vi "getWaypoints.vi"(8 "Error In":errorcluster, 10 "NotifierReff 2":T1, 11 "RoundBouy in":refnum<class "RoundBouy.lvclass">) -> (0 "Error Out":errorcluster, 2 "Waypoint Array":refnum<class "Waypoint.lvclass">[](array[class]), 3 "RoundBouy out":refnum<class "RoundBouy.lvclass">)   [LabVIEW 2013, in "RoundBouy.lvclass"]
doc: "Generate and get the critical waypoints. In this case, at least two are generated, with a third dependent on where the next mission is. These also depend on which direction around the buoy the boat is going."
uses:
  RoundBouy.lvclass
  Waypoint/Waypoint.lvclass
  Data/TypeDefs/Notifiers.ctl
  Data/TypeDefs/UTM Location.ctl
  Data/TypeDefs/Sail Set Suggestions.ctl
  Data/TypeDefs/Rudder Set Suggestions.ctl
  Data/TypeDefs/OverrideInformation.ctl
  Data/TypeDefs/OverrideMode.ctl
  Data/TypeDefs/MotorSetup.ctl
  Data/TypeDefs/DynamixelSetupInfo.ctl
  Data/TypeDefs/AirmarStatus.ctl
  Data/TypeDefs/HardwareOnline.ctl
  Data/TypeDefs/DynamixelCycleTracker.ctl
  Data/TypeDefs/RC Input Values.ctl
  GenericMission/GenericMission.lvclass
  RoundBouy.lvclass/RoundBouy.ctl
  <vilib>/Analysis/coordinate.llb/2D Cartesian Coordinate Shift (Scalar).vi
  <vilib>/Analysis/coordinate.llb/2D Cartesian Coordinate Rotation (Scalar).vi
  <vilib>/Analysis/NI_AALPro.lvlib
panel:
  out "Mission X":dbl
  out "Mission Y":dbl
  out "wp1 Y":dbl
  out "wp1 X":dbl
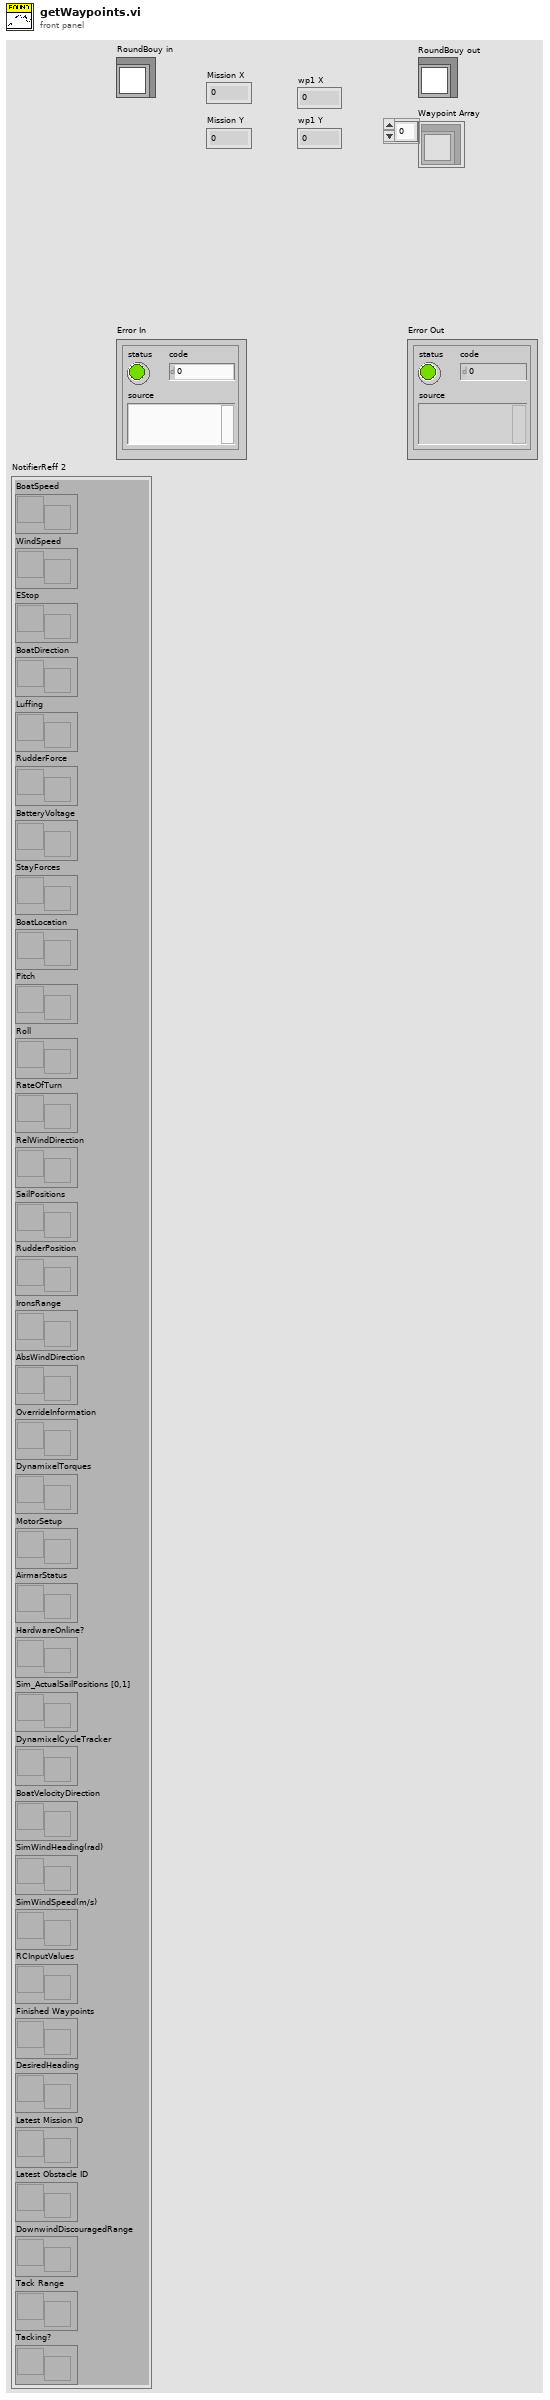
[diagram p1: front panel]
types:
  T1 = typedef "Notifiers.ctl" = cluster{"BoatSpeed":refnum<notifier>, "WindSpeed":refnum<notifier>, "EStop":refnum<notifier>, "BoatDirection":refnum<notifier>, "Luffing":refnum<notifier>, "RudderForce":refnum<notifier>, "BatteryVoltage":refnum<notifier>, "StayForces":refnum<notifier>, "BoatLocation":refnum<notifier>, "Pitch":refnum<notifier>, "Roll":refnum<notifier>, "RateOfTurn":refnum<notifier>, "RelWindDirection":refnum<notifier>, "SailPositions":refnum<notifier>, "RudderPosition":refnum<notifier>, "IronsRange":refnum<notifier>, "AbsWindDirection":refnum<notifier>, "OverrideInformation":refnum<notifier>, "DynamixelTorques":refnum<notifier>, "MotorSetup":refnum<notifier>, "AirmarStatus":refnum<notifier>, "HardwareOnline?":refnum<notifier>, "Sim_ActualSailPositions [0,1]":refnum<notifier>, "DynamixelCycleTracker":refnum<notifier>, "BoatVelocityDirection":refnum<notifier>, "SimWindHeading(rad)":refnum<notifier>, "SimWindSpeed(m/s)":refnum<notifier>, "RCInputValues":refnum<notifier>, "Finished Waypoints":refnum<notifier>, "DesiredHeading":refnum<notifier>, "Latest Mission ID":refnum<notifier>, "Latest Obstacle ID":refnum<notifier>, "DownwindDiscouragedRange":refnum<notifier>, "Tack Range":refnum<notifier>, "Tacking?":refnum<notifier>}
  T2 = typedef "UTM Location.ctl" = cluster{"UTM Zone":dbl, "Hemisphere":enum16{"North", "South"}, "East":dbl, "North":dbl}
  T3 = typedef "MissionTypeControl.ctl" = enum16{"Idle at Point", "Drive to Waypoint", "Round Buoy to Port", "Round Buoy to Starboard", "Pass Between Buoys", "Station Keeping"}
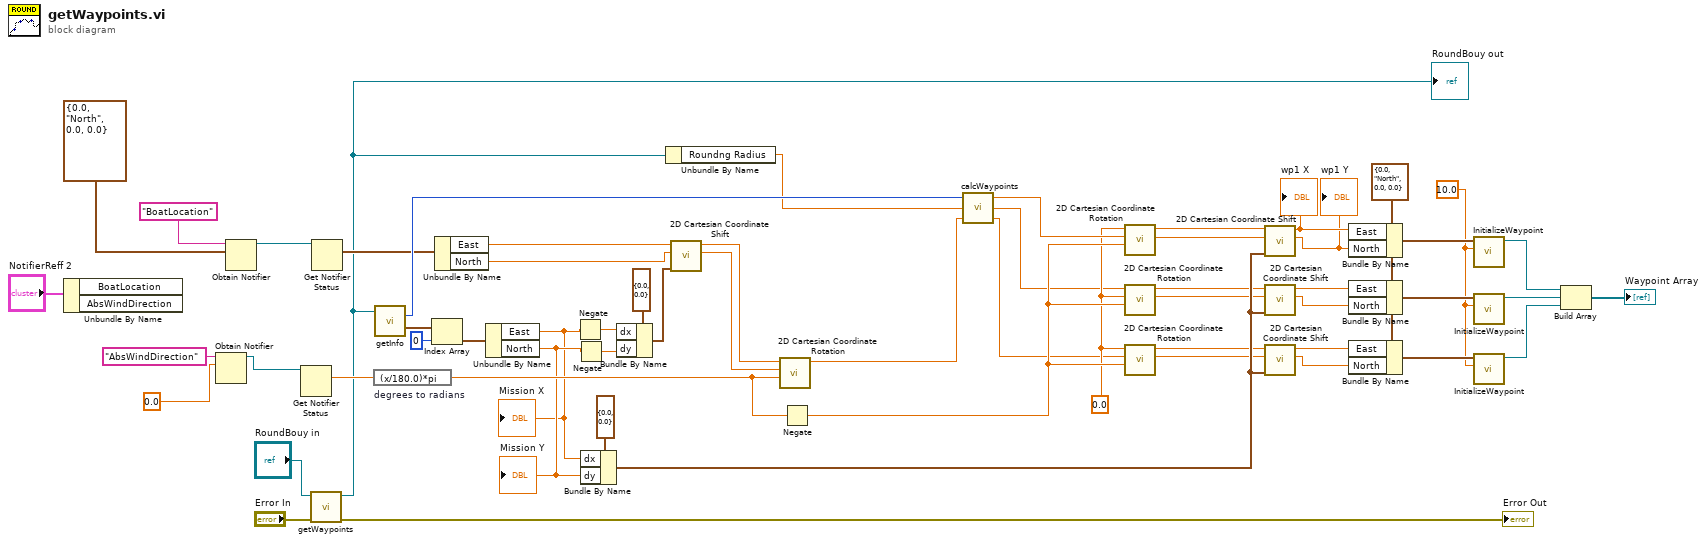
[diagram p0: block diagram]
diagram:
  w12 = 10.0
  w40 = 0.0 ("East")
  w44 = T2 {"UTM Zone"=0.0, "Hemisphere"=enum."North", "East"=0.0, "North"=0.0} ("Coords")
  n1 = Unbundle By Name("NotifierReff 2") -> ()  [unwired: 2 out]
  n2 = Obtain Notifier(name (unnamed)="AbsWindDirection", notification data type=0.0 ("latest notification")) -> (notifier out=w13:refnum<notifier>)  [unwired: 2 in, 2 out]
  n3 = Obtain Notifier(name (unnamed)="BoatLocation", notification data type=T2 {"UTM Zone"=0.0, "Hemisphere"=enum."North", "East"=0.0, "North"=0.0} ("latest notification")) -> (notifier out=w19:refnum<notifier>)  [unwired: 2 in, 2 out]
  n4 = Get Notifier Status(notifier=w13) -> (current notification=w11:dbl)  [unwired: 1 in, 4 out]
  n5 = call-parent "getWaypoints.vi"("Error In"="Error In", "GenericMission in"="RoundBouy in") -> ("Error Out"=→"Error Out":errorcluster, "GenericMission out"=w2:refnum<class "RoundBouy.lvclass">)  [unwired: 7 in, 1 out]
  "RoundBouy out" <- w2
  n6 = Get Notifier Status(notifier=w19) -> (current notification=w16:T2)  [unwired: 1 in, 4 out]
  n7 = expression code="(x/180.0)*pi" "degrees to radians"(w11) -> (w10:dbl)
  n8 = call-dynamic "getInfo.vi"("GenericMission in"=w2) -> ("Mission Type"=w43:T3, "Points of Interest"=w55:T2[])  [unwired: 6 in, 7 out]
  n9 = Index Array(array=w55, index=0) -> (element=w53:T2)
  n10 = Unbundle By Name(w16) -> ("East"=w8:dbl, "North"=w9:dbl)
  n11 = Unbundle By Name(w53) -> ("East"=w3:dbl, "North"=w4:dbl)
  "Mission Y" <- w4
  "Mission X" <- w3
  n12 = Negate(x=w3) -> (-x=w6:dbl)
  n13 = Negate(x=w4) -> (-x=w5:dbl)
  n14 = Bundle By Name(cluster=cluster{"dx":dbl, "dy":dbl} {"dx"=0.0, "dy"=0.0} ("shift"), "dx"=w3, "dy"=w4) -> (w36:cluster{"dx":dbl, "dy":dbl})
  n15 = Bundle By Name(cluster=cluster{"dx":dbl, "dy":dbl} {"dx"=0.0, "dy"=0.0} ("shift"), "dx"=w6, "dy"=w5) -> (w51:cluster{"dx":dbl, "dy":dbl})
  n16 = Unbundle By Name(w2) -> ("Roundng Radius"=w1:dbl)
  n17 = call-poly <vilib>:"2D Cartesian Coordinate Shift.vi"("shift"=w51, "y"=w9, "x"=w8) -> ("y out"=w50:dbl, "x out"=w49:dbl)  [unwired: 6 in, 1 out]
  n18 = call-poly <vilib>:"2D Cartesian Coordinate Rotation.vi"("theta"=w10, "y"=w50, "x"=w49) -> ("x out"=w7:dbl)  [unwired: 6 in, 2 out]
  n19 = Negate(x=w10) -> (-x=w41:dbl)
  n20 = call "calcWaypoints.vi"("boat x"=w7, "Clearance"=w1, "Mission Type"=w43) -> ("y 3"=w38:dbl, "x 2"=w39:dbl, "y 1"=w42:dbl)
  n21 = call-poly <vilib>:"2D Cartesian Coordinate Rotation.vi"("theta"=w41, "y"=w42, "x"=w40) -> ("y out"=w34:dbl, "x out"=w35:dbl)  [unwired: 6 in, 1 out]
  n22 = call-poly <vilib>:"2D Cartesian Coordinate Rotation.vi"("theta"=w41, "y"=w40, "x"=w39) -> ("y out"=w32:dbl, "x out"=w33:dbl)  [unwired: 6 in, 1 out]
  n23 = call-poly <vilib>:"2D Cartesian Coordinate Rotation.vi"("theta"=w41, "y"=w38, "x"=w40) -> ("y out"=w30:dbl, "x out"=w31:dbl)  [unwired: 6 in, 1 out]
  n24 = call-poly <vilib>:"2D Cartesian Coordinate Shift.vi"("shift"=w36, "y"=w34, "x"=w35) -> ("y out"=w28:dbl, "x out"=w29:dbl)  [unwired: 6 in, 1 out]
  "wp1 X" <- w29
  "wp1 Y" <- w28
  n25 = call-poly <vilib>:"2D Cartesian Coordinate Shift.vi"("shift"=w36, "y"=w32, "x"=w33) -> ("y out"=w26:dbl, "x out"=w27:dbl)  [unwired: 6 in, 1 out]
  n26 = call-poly <vilib>:"2D Cartesian Coordinate Shift.vi"("shift"=w36, "y"=w30, "x"=w31) -> ("y out"=w24:dbl, "x out"=w25:dbl)  [unwired: 6 in, 1 out]
  n27 = Bundle By Name(cluster=w44, "East"=w29, "North"=w28) -> (w23:T2)
  n28 = Bundle By Name(cluster=w44, "East"=w27, "North"=w26) -> (w22:T2)
  n29 = Bundle By Name(cluster=w44, "East"=w25, "North"=w24) -> (w21:T2)
  n30 = call "InitializeWaypoint.vi"("Tolerance (meters?) (0)"=w12, "Coords"=w23) -> ("Waypoint Out"=w48:refnum<class "Waypoint.lvclass">)  [unwired: 9 in]
  n31 = call "InitializeWaypoint.vi"("Tolerance (meters?) (0)"=w12, "Coords"=w22) -> ("Waypoint Out"=w46:refnum<class "Waypoint.lvclass">)  [unwired: 9 in]
  n32 = call "InitializeWaypoint.vi"("Tolerance (meters?) (0)"=w12, "Coords"=w21) -> ("Waypoint Out"=w47:refnum<class "Waypoint.lvclass">)  [unwired: 9 in]
  n33 = Build Array(w48, w46, w47) -> (→"Waypoint Array":refnum<class "Waypoint.lvclass">[])
